vi "LINAKSetNLaunch.vi"(7 "LINAKAddresses":u8[](array[numeric]), 8 "error in (no error)":errorcluster, 10 "AbsRequests":dbl[](array[numeric])) -> (0 "error out":errorcluster)   [LabVIEW 2021]
uses:
  LINAKUTIL.ctl
  Anemometry/Anemometry Sub Vis/Globals/Preference_global.vi
panel:
  out "x":i32=2
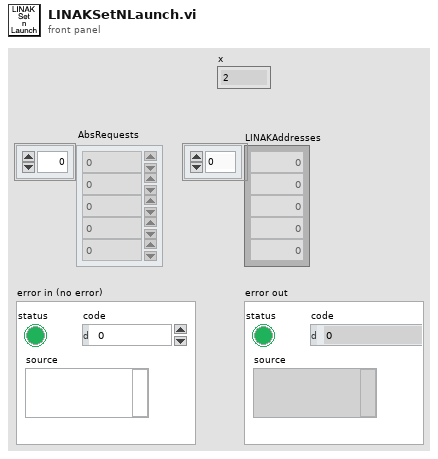
[diagram p1: front panel]
types:
  T1 = typedef "LINAKUTIL.ctl" = enum16{"Read", "ReadTarget", "WriteTarget", "SingleGo", "GlobalGo", "SafetySet", "WriteReadGo", "STOP"}
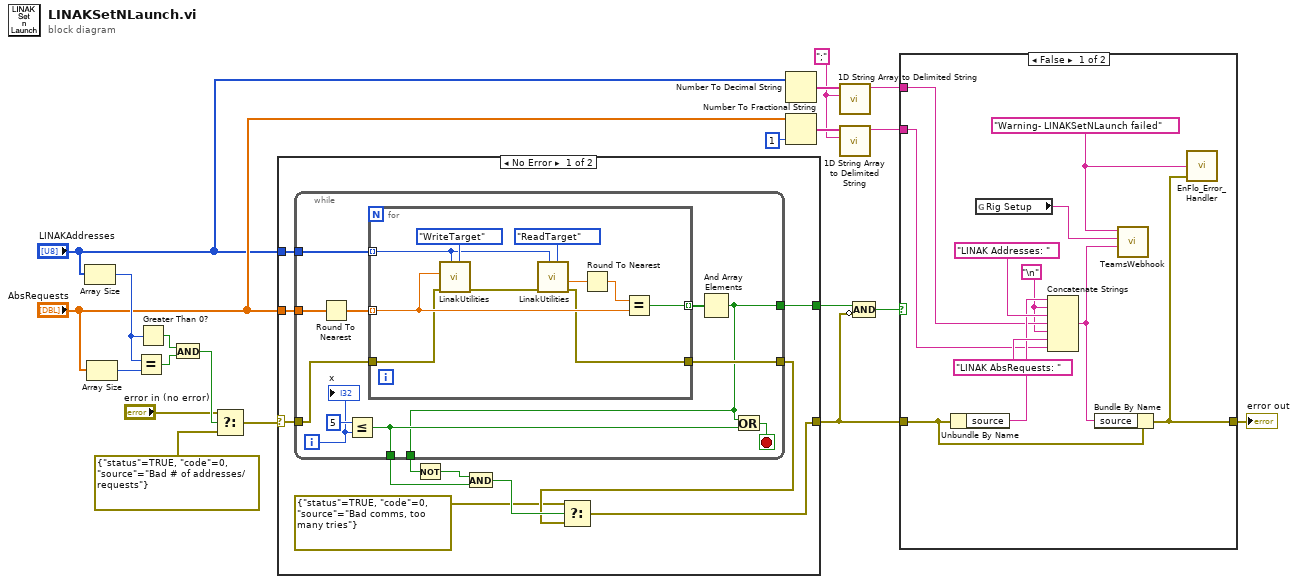
[diagram p0: block diagram]
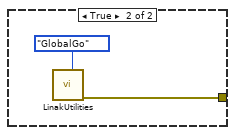
[diagram p2: hidden frame]
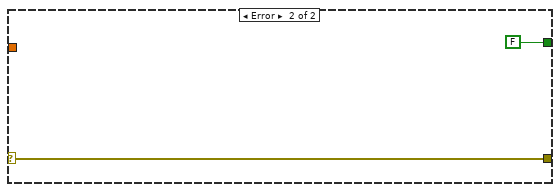
[diagram p3: hidden frame]
diagram:
  w1 = ";" ("delimiter")
  n1 = Array Size(array="LINAKAddresses") -> (size(s)=w12:i32)
  n2 = Array Size(array="AbsRequests") -> (size(s)=w19:i32)
  n3 = Equal?(x=w12, y=w19) -> (x = y?=w18:bool)
  n4 = Greater Than 0?(x=w12) -> (x > 0?=w17:bool)
  n5 = And(x=w17, y=w18) -> (x .and. y?=w16:bool)
  n6 = Select(t="error in (no error)", s=w16, f=errorcluster {"status"=TRUE, "code"=0, "source"="Bad # of addresses/requests"} ("t")) -> (s? t:f=w13:errorcluster)
  n7 = case shown="No Error" w13 {
    selector: w13 -> [w29 w53]
    tunnel: "AbsRequests" -> [w31 _]
    tunnel: "LINAKAddresses" -> [w30 _]
    tunnel: [w28 FALSE] -> w20
    tunnel: [w21 w53] -> w10
    frame No Error {
      n8 = while {
        tunnel: w31 -> [w41]
        tunnel: w30 -> [w40]
        tunnel: w29 -> [w37]
        tunnel: [w39] -> w23
        tunnel: [w34] -> w28
        tunnel: [w35] -> w27
        tunnel: [w34] -> w26
        i -> [w32]
        stop <- w36 stop-if-true
        n9 = Round To Nearest(number=w41) -> (nearest integer value=w42:dbl[])
        n10 = Less Or Equal?(x=5, y=w32) -> (x <= y?=w35:bool)
        n11 = for {
          tunnel: w42 -> [w45] mode=indexing
          tunnel: [w52] -> w38 mode=indexing
          tunnel: w40 -> [w48] mode=indexing
          tunnel: w37 -> [w43]
          tunnel: [w44] -> w39
          n12 = call "LinakUtilities.vi"("LinakUtil"=LINAKUTIL."WriteTarget", "Linak Address"=w48, "error in (no error)"=w43, "Request(mm)"=w45) -> ("error out"=w47:errorcluster)  [unwired: 4 in, 3 out]
          n13 = call "LinakUtilities.vi"("LinakUtil"=LINAKUTIL."ReadTarget", "Linak Address"=w48, "error in (no error)"=w47) -> ("error out"=w44:errorcluster, "Target(mm)"=w46:dbl)  [unwired: 5 in, 2 out]
          n14 = Round To Nearest(number=w46) -> (nearest integer value=w51:dbl)
          n15 = Equal?(x=w51, y=w45) -> (x = y?=w52:bool)
        }
        n16 = And Array Elements(Boolean array=w38) -> (logical AND=w34:bool)
        n17 = Or(x=w34, y=w35) -> (x .or. y?=w36:bool)
        "x" <- w32
      }
      n18 = Not(x=w26) -> (.not. x?=w25:bool)
      n19 = And(x=w25, y=w27) -> (x .and. y?=w24:bool)
      n20 = Select(t=errorcluster {"status"=TRUE, "code"=0, "source"="Bad comms, too many tries"}, s=w24, f=w23) -> (s? t:f=w21:errorcluster)
    }
    frame Error {
    }
  }
  n21 = Number To Decimal String(number="LINAKAddresses") -> (decimal integer string=w4:string[])  [unwired: 1 in]
  n22 = Number To Fractional String(number="AbsRequests", precision (6)=i16 1) -> (F-format string=w7:string[])  [unwired: 2 in]
  n23 = call <vilib>:"1D String Array to Delimited String.vi"("delimiter"=w1, "string array"=w4) -> ("delimited string"=w2:string)  [unwired: 9 in]
  n24 = call <vilib>:"1D String Array to Delimited String.vi"("delimiter"=w1, "string array"=w7) -> ("delimited string"=w5:string)  [unwired: 9 in]
  n25 = Compound Arithmetic op=AND(w20, invert w10) -> (w11:bool)
  n26 = case shown="False" w11 {
    tunnel: w10 -> [w62 _]
    tunnel: [w61 w66] -> w9
    tunnel: w5 -> [w60 _]
    tunnel: w2 -> [w59 _]
    frame False {
      w58 = "\n"
      w57 = "Warning- LINAKSetNLaunch failed" ("Error Type")
      n27 = Unbundle By Name(w62) -> ("source"=w63:string)
      n28 = global read "Preference_global.vi" "Rig Setup"() -> (w55:string)
      n29 = Concatenate Strings(w63, w58, "LINAK Addresses: ", w59, w58, "LINAK AbsRequests: ", w60) -> (w56:string)
      n30 = Bundle By Name(cluster=w62, "source"=w56) -> (w61:errorcluster)
      n31 = call "TeamsWebhook.vi"("Source"=w57, "Type"=w55, "Reason"=w56) -> ()  [unwired: 2 in, 1 out]
      n32 = call "EnFlo_Error_Handler.vi"("error in (no error)"=w61, "Error Type"=w57) -> ()  [unwired: 2 in, 2 out]
    }
    frame True {
      n33 = call "LinakUtilities.vi"("LinakUtil"=LINAKUTIL."GlobalGo") -> ("error out"=w66:errorcluster)  [unwired: 7 in, 3 out]
    }
  }
  "error out" <- w9
